vi "Read Driver Joystick.vi"(11 "Driver Joystick":T1) -> ()   [LabVIEW 2019]
uses:
  <vilib>/Rock Robotics/WPI/Joystick/WPI_JoystickDevRef.ctl
  <vilib>/Rock Robotics/WPI/Joystick/WPI_JoystickDeviceEnum.ctl
  Framework/Robot Global Data.vi
  Controls/Joystick Mini Sticks.ctl
  Controls/Joystick Buttons.ctl
panel:
  # "READ DRIVER JOYSTICK"
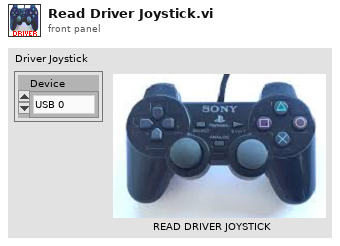
[diagram p1: front panel]
types:
  T1 = typedef "WPI_JoystickDevRef.ctl" = cluster{"Device":T2}
  T2 = typedef "WPI_JoystickDeviceEnum.ctl" = enum16{"USB 0", "USB 1", "USB 2", "USB 3", "USB 4", "USB 5"}
  T3 = typedef "Joystick Buttons.ctl" = enum16{"Triangle 0", "Circle 1", "X 2", "Square 3", "Left Button 4", "Right Button 5", "Left Trigger 6", "Right Trigger 7"}
  T4 = typedef "Joystick Mini Sticks.ctl" = enum16{"Left Stick 0: X Axis", "Left Stick 1: Y Axis", "Right Stick 2: Z Axis", "Right Stick 3: Z Rotates"}
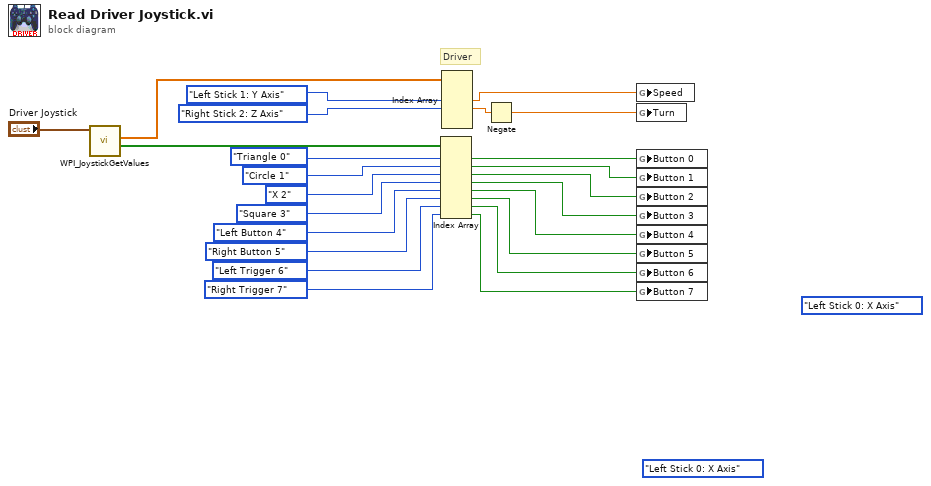
[diagram p0: block diagram]
diagram:
  (unwired) Joystick_Mini_Sticks."Left Stick 0: X Axis" ("Joystick Mini Sticks")
  (unwired) Joystick_Mini_Sticks."Left Stick 0: X Axis" ("Joystick Mini Sticks")
  # "Driver"
  n1 = call <vilib>:"WPI_JoystickGetValues.vi"("JoystickDevRef"="Driver Joystick") -> ("Buttons"=w23:bool[], "Axes"=w22:dbl[])  [unwired: 6 in, 3 out]
  n2 = Index Array(array=w23, index #1=Joystick_Buttons."Triangle 0" ("Joystick Buttons"), index #2=Joystick_Buttons."Circle 1" ("Joystick Buttons"), index #3=Joystick_Buttons."X 2" ("Joystick Buttons"), index #4=Joystick_Buttons."Square 3" ("Joystick Buttons"), index #5=Joystick_Buttons."Left Button 4" ("Joystick Buttons"), index #6=Joystick_Buttons."Right Button 5" ("Joystick Buttons"), index #7=Joystick_Buttons."Left Trigger 6" ("Joystick Buttons"), index #8=Joystick_Buttons."Right Trigger 7" ("Joystick Buttons")) -> (element #1=w24:bool, element #2=w21:bool, element #3=w20:bool, element #4=w16:bool, element #5=w19:bool, element #6=w18:bool, element #7=w17:bool, element #8=w15:bool)
  n3 = Index Array(array=w22, index #2=Joystick_Mini_Sticks."Left Stick 1: Y Axis" ("Joystick Mini Sticks"), index #3=Joystick_Mini_Sticks."Right Stick 2: Z Axis" ("Joystick Mini Sticks")) -> (element #2=w11:dbl, element #3=w12:dbl)  [unwired: 3 in, 3 out]
  n4 = Negate(x=w12) -> (-x=w14:dbl)
  n5 = global write "Robot Global Data.vi" "Speed"(w11) -> ()
  n6 = global write "Robot Global Data.vi" "Turn"(w14) -> ()
  n7 = global write "Robot Global Data.vi" "Button 0"(w24) -> ()
  n8 = global write "Robot Global Data.vi" "Button 1"(w21) -> ()
  n9 = global write "Robot Global Data.vi" "Button 2"(w20) -> ()
  n10 = global write "Robot Global Data.vi" "Button 3"(w16) -> ()
  n11 = global write "Robot Global Data.vi" "Button 4"(w19) -> ()
  n12 = global write "Robot Global Data.vi" "Button 5"(w18) -> ()
  n13 = global write "Robot Global Data.vi" "Button 6"(w17) -> ()
  n14 = global write "Robot Global Data.vi" "Button 7"(w15) -> ()
